vi "OverlayOval.vi"   [LabVIEW 2024, in "OpenLvVision_Overlays.lvlib"]
doc: "Overlays an oval on top of an image."
uses:
  OpenLvVision_Overlays.lvlib
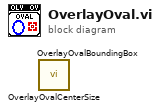
[diagram p0: block diagram]
diagram:
  n1 = call "OverlayOvalCenterSize.vi"() -> ()  [unwired: 10 in, 2 out]
  n2 = call "OverlayOvalBoundingBox.vi"() -> ()  [unwired: 10 in, 2 out]
